vi "New MultiBluePlot.vi"(8 "error in (no error)":errorcluster, 9 "Multi Plot Init Options":T1={"config file start path"=path "", "Layout"=[{"Plot Number"=1, "Plot Bounds (%)"={"Left (%)"=0.0, "Top (%)"=0.0, "Right (%)"=50.0, "Bottom (%)"=50.0}}, {"Plot Number"=2, "Plot Bounds (%)"={"Left (%)"=50.0, "Top (%)"=0.0, "Right (%)"=100.0, "Bottom (%)"=50.0}}, {"Plot Number"=3, "Plot Bounds (%)"={"Left (%)"=0.0, "Top (%)"=50.0, "Right (%)"=50.0, "Bottom (%)"=100.0}}, {"Plot Number"=4, "Plot Bounds (%)"={"Left (%)"=50.0, "Top (%)"=50.0, "Right (%)"=100.0, "Bottom (%)"=100.0}}]} {"Layout"."Plot Bounds (%)"."Bottom (%)" format="%.2f"; "Layout"."Plot Bounds (%)"."Top (%)" format="%.2f"; "Layout"."Plot Bounds (%)"."Right (%)" format="%.2f"; "Layout"."Plot Bounds (%)"."Left (%)" format="%.2f"}, 11 "RocketPlotPanel":refnum<class "RocketPlotPanel.lvclass">) -> (0 "error out":errorcluster, 3 "MultiPlotPanel (type)":refnum<class "MultiRocketPlotPanel.lvclass">)   [LabVIEW 2021, in "MultiRocketPlotPanel.lvclass"]
uses:
  MultiRocketPlotPanel.lvclass
  Init options.ctl
  SubVIs/Window Position and plot number.ctl
  SubVIs/Window Position.ctl
  <userlib>/bjustice/RocketPlot/Classes/RocketPlotPanel/RocketPlotPanel.lvclass
  <userlib>/bjustice/RocketPlot/TypeDefs/panel mode.ctl
  <userlib>/bjustice/RocketPlot/Classes/RocketPlotPanel/RocketPlotPanel.lvclass/RocketPlotPanel.ctl
  MultiRocketPlotPanel.lvclass/MultiRocketPlotPanel.ctl
  <userlib>/bjustice/RocketPlot/Classes/RocketPlotPanel/Write panel mode.vi
  <userlib>/bjustice/RocketPlot/RocketPlot.lvlib
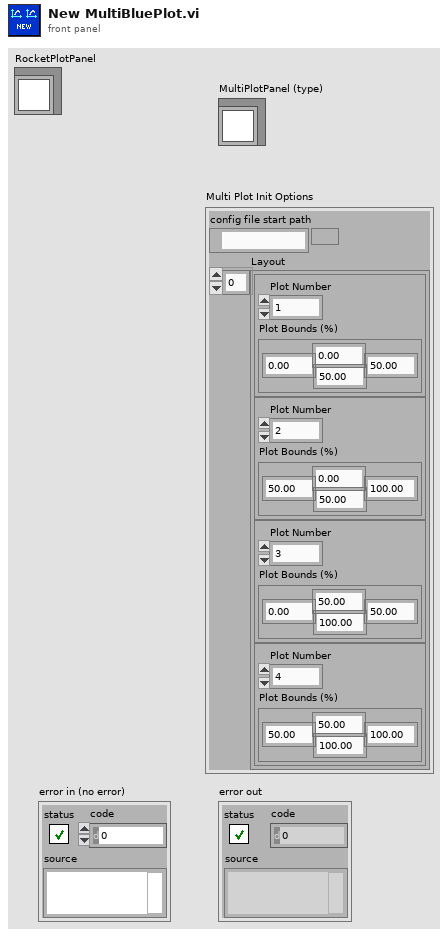
[diagram p1: front panel]
types:
  T1 = typedef "MultiRocketPlotPanel.lvclass/Init options.ctl" = cluster{"config file start path":path, "Layout":T2[]}
  T2 = typedef "MultiRocketPlotPanel.lvclass/Window Position and plot number.ctl" = cluster{"Plot Number":i32, "Plot Bounds (%)":T3}
  T3 = typedef "MultiRocketPlotPanel.lvclass/Window Position.ctl" = cluster{"Left (%)":dbl, "Top (%)":dbl, "Right (%)":dbl, "Bottom (%)":dbl}
  T4 = typedef "RocketPlot.lvlib/panel mode.ctl" = enum16{"1PLOT", "MPLOT"}
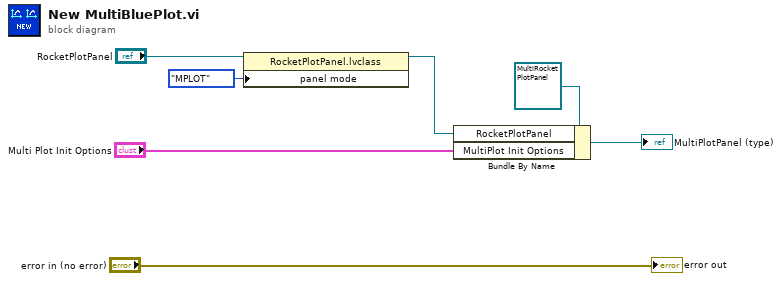
[diagram p0: block diagram]
diagram:
  n1 = property class="RocketPlotPanel.lvclass"(reference="RocketPlotPanel", "panel mode"=panel_mode."MPLOT") -> (reference out=w1:refnum<class "RocketPlotPanel.lvclass">)  [unwired: 1 in, 1 out]
  n2 = Bundle By Name(cluster=refnum<class "MultiRocketPlotPanel.lvclass"> refnum ("MultiPlotPanel out"), "RocketPlotPanel"=w1, "MultiPlot Init Options"="Multi Plot Init Options") -> (→"MultiPlotPanel (type)":refnum<class "MultiRocketPlotPanel.lvclass">)
  "error out" <- "error in (no error)"
